vi "Set Power Array Parameters.vi"(8 "error in (no error)":errorcluster, 10 "Step In":refnum<k7>, 11 "ModSweep in":refnum<class "Power Sweep.lvclass">) -> (0 "error out":errorcluster, 2 "Step Out":refnum<k7>, 3 "ModSweep out":refnum<class "Power Sweep.lvclass">)   [LabVIEW 2018, in "Power Sweep.lvlib" / "Power Sweep.lvclass"]
uses:
  Power Sweep.lvclass
  Power Sweep.lvclass/Power Sweep.ctl
  Plugins/Measurement Interface.lvlibp/Measurement Interface.lvclass
  C:/Sequence Automation/Plugins/Measurement Interface.lvlibp/Measurement Interface.lvclass
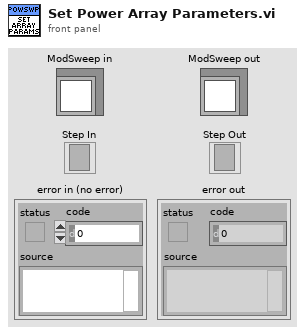
[diagram p1: front panel]
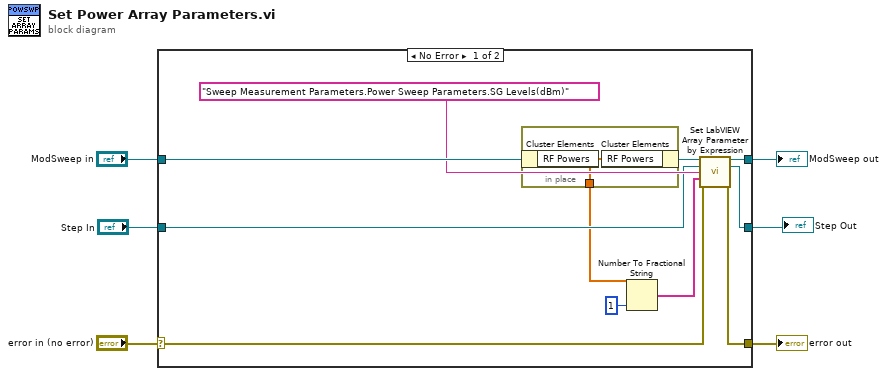
[diagram p0: block diagram]
diagram:
  n1 = case shown="No Error" "error in (no error)" {
    selector: "error in (no error)" -> [w17 w21]
    tunnel: [w15 w21] -> w5
    tunnel: [w7 w20] -> w3
    tunnel: "ModSweep in" -> [w16 w20]
    tunnel: "Step In" -> [w13 w19]
    tunnel: [w12 w19] -> w1
    frame No Error {
      n2 = in-place {
        in-place-border: [w18] -> w11
        n3 = in-place-cluster #1(w16) -> ("RF Powers"=w18:dbl[])
        n4 = in-place-cluster #1("RF Powers"=w18) -> (w8:refnum<class "Power Sweep.lvclass">)
      }
      n5 = Number To Fractional String(number=w11, precision (6)=i16 1) -> (F-format string=w10:string[])  [unwired: 2 in]
      n6 = call "Set LabVIEW Array Parameter by Expression.vi"("Measurement Interface in"=w8, "Step In"=w13, "LabVIEW Parameter to Set"="Sweep Measurement Parameters.Power Sweep Parameters.SG Levels(dBm)" ("lookupString"), "Array of Expresssions"=w10, "error in (no error)"=w17) -> ("Measurement Interface out"=w7:refnum<class "Power Sweep.lvclass">, "Step Out"=w12:refnum<k7>, "error out"=w15:errorcluster)  [unwired: 8 in]
    }
    frame Error {
    }
  }
  "error out" <- w5
  "ModSweep out" <- w3
  "Step Out" <- w1
